vi "Labview_Database_write.vi"() -> ()   [LabVIEW 2012]
uses:
  <vilib>/addons/database/NI_Database_API.lvlib
  <vilib>/addons/database/Connection.llb/DB Tools Open Connec (Path).vi
  <vilib>/FieldPoint/Polymorphic Write.llb/FP Write (Float -IO).vi
  <vilib>/FieldPoint/Polymorphic Read.llb/FP Read (Float -IO).vi
  LabView ESIII/LabView ESIII/try.llb/Control 2.ctl
panel:
  out "current time":timestamp
  out "cFP-AI-112":dbl(graph)
  out "cFP-DO-401":dbl(graph)
  in  "Digital Output Switch":bool
  in  "sample data":T1={"String"="This is a test string", "Numeric"=101, "Numeric 2"=3.14} {"Numeric 2" format="%.2f"}
  out "tables":T2[](array[typedef])
  in  "stop":bool
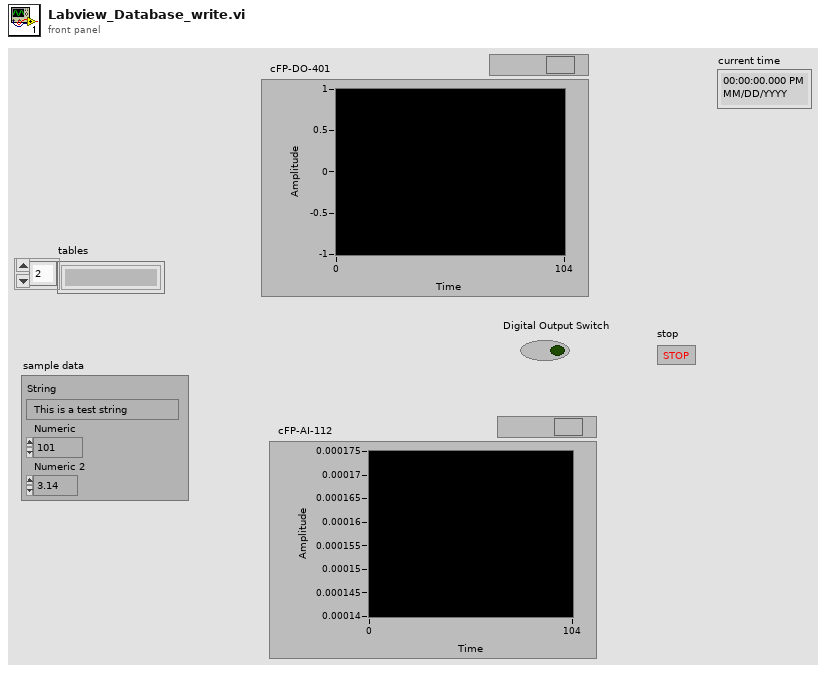
[diagram p1: front panel]
types:
  T1 = cluster{"String":string, "Numeric":i32, "Numeric 2":dbl}
  T2 = typedef "Control 2.ctl" = string
  T3 = typedef "NI_Database_API.lvlib/Conn ObjectReference.ctl" = refnum<k1>
  T4 = cluster{"date/time string":string, "value":dbl, "value":dbl}
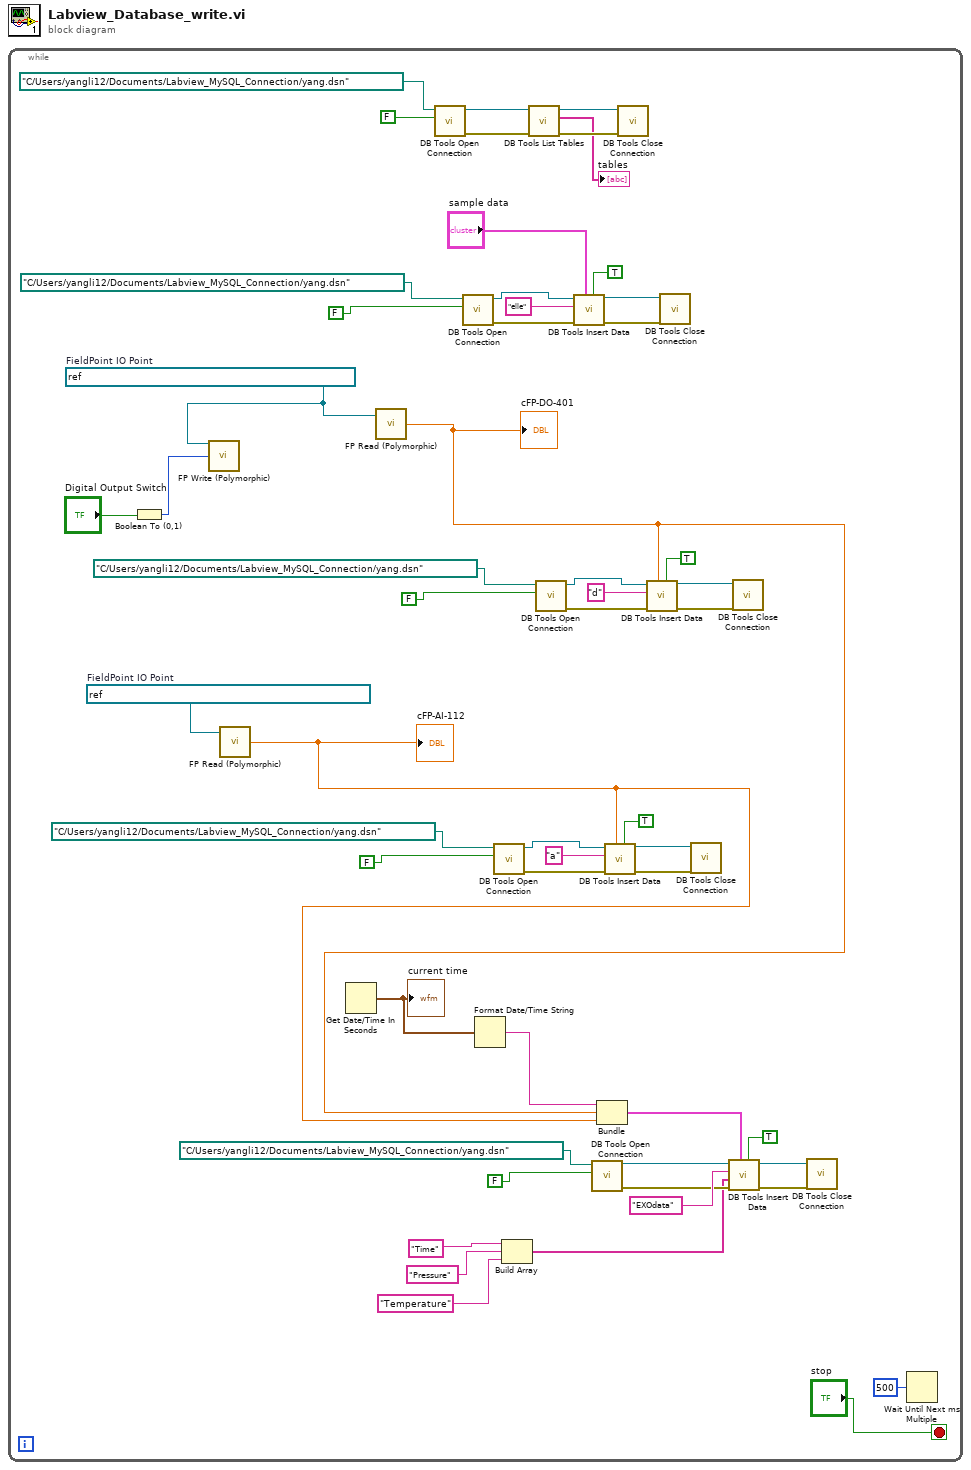
[diagram p0: block diagram]
diagram:
  n1 = while {
    stop <- "stop" stop-if-true
    w26 = refnum<k21> "FieldPoint\\Loomis434\\cFP-AI-112 @5\\Channel 0"  # FieldPoint IO Point
    w27 = refnum<k21> "FieldPoint\\Loomis434\\cFP-DO-401 @4\\Channel 0"  # FieldPoint IO Point
    n2 = Boolean To (0,1)(Boolean="Digital Output Switch") -> (0, 1=w28:i16)
    n3 = call-poly <vilib>:"FP Write (Polymorphic).vi"("FieldPoint IO Point In"=w27, "value"=w28) -> ()  [unwired: 11 in, 3 out]
    n4 = call-poly <vilib>:"FP Read (Polymorphic).vi"("FieldPoint IO Point In"=w26) -> ("value"=w10:dbl)  [unwired: 11 in, 3 out]
    "cFP-AI-112" <- w10
    n5 = Get Date/Time In Seconds() -> (seconds since 1Jan1904=w3:timestamp)
    "current time" <- w3
    n6 = call-poly <vilib>:"FP Read (Polymorphic).vi"("FieldPoint IO Point In"=w27) -> ("value"=w11:dbl)  [unwired: 11 in, 3 out]
    "cFP-DO-401" <- w11
    n7 = call-poly <vilib>:"DB Tools Open Connection.vi"("prompt? (F)"=FALSE, "connection information"=path "C:/Users/yangli12/Documents/Labview_MySQL_Connection/yang.dsn") -> ("error out"=w46:errorcluster, "connection reference"=w49:T3)  [unwired: 6 in]
    n8 = call-poly <vilib>:"DB Tools Open Connection.vi"("prompt? (F)"=FALSE, "connection information"=path "C:/Users/yangli12/Documents/Labview_MySQL_Connection/yang.dsn") -> ("error out"=w42:errorcluster, "connection reference"=w43:T3)  [unwired: 6 in]
    n9 = Format Date/Time String(seconds (now)=w3) -> (date/time string=w4:string)  [unwired: 2 in]
    n10 = call-poly <vilib>:"DB Tools Open Connection.vi"("prompt? (F)"=FALSE, "connection information"=path "C:/Users/yangli12/Documents/Labview_MySQL_Connection/yang.dsn") -> ("error out"=w20:errorcluster, "connection reference"=w21:T3)  [unwired: 6 in]
    n11 = Build Array("Time" ("table"), "Pressure" ("table"), "Temperature" ("table")) -> (w5:string[])
    n12 = call <vilib>:"DB Tools List Tables.vi"("error in (no error)"=w46, "connection reference"=w49) -> ("error out"=w53:errorcluster, "tables"=→"tables":string[], "connection reference out"=w54:T3)  [unwired: 3 in]
    n13 = call-poly <vilib>:"DB Tools Open Connection.vi"("prompt? (F)"=FALSE, "connection information"=path "C:/Users/yangli12/Documents/Labview_MySQL_Connection/yang.dsn") -> ("error out"=w32:errorcluster, "connection reference"=w33:T3)  [unwired: 6 in]
    n14 = call <vilib>:"DB Tools Insert Data.vi"("create table? (F)"=TRUE, "data"="sample data", "error in (no error)"=w42, "table"="elle", "connection reference"=w43) -> ("error out"=w47:errorcluster, "connection reference out"=w48:T3)  [unwired: 5 in]
    n15 = call-poly <vilib>:"DB Tools Open Connection.vi"("prompt? (F)"=FALSE, "connection information"=path "C:/Users/yangli12/Documents/Labview_MySQL_Connection/yang.dsn") -> ("error out"=w12:errorcluster, "connection reference"=w13:T3)  [unwired: 6 in]
    n16 = Bundle("date/time string"=w4, "value"=w11, "value"=w10) -> (w9:T4)  [unwired: 1 in]
    n17 = call <vilib>:"DB Tools Insert Data.vi"("create table? (F)"=TRUE, "data"=w10, "error in (no error)"=w20, "table"="a", "connection reference"=w21) -> ("error out"=w24:errorcluster, "connection reference out"=w25:T3)  [unwired: 5 in]
    n18 = call <vilib>:"DB Tools Close Connection.vi"("error in (no error)"=w53, "connection reference"=w54) -> ()  [unwired: 5 in, 1 out]
    n19 = call <vilib>:"DB Tools Insert Data.vi"("create table? (F)"=TRUE, "data"=w11, "error in (no error)"=w32, "table"="d", "connection reference"=w33) -> ("error out"=w36:errorcluster, "connection reference out"=w37:T3)  [unwired: 5 in]
    n20 = call <vilib>:"DB Tools Close Connection.vi"("error in (no error)"=w47, "connection reference"=w48) -> ()  [unwired: 5 in, 1 out]
    n21 = call <vilib>:"DB Tools Close Connection.vi"("error in (no error)"=w24, "connection reference"=w25) -> ()  [unwired: 5 in, 1 out]
    n22 = call <vilib>:"DB Tools Insert Data.vi"("create table? (F)"=TRUE, "data"=w9, "error in (no error)"=w12, "columns"=w5, "table"="EXOdata", "connection reference"=w13) -> ("error out"=w1:errorcluster, "connection reference out"=w2:T3)  [unwired: 4 in]
    n23 = call <vilib>:"DB Tools Close Connection.vi"("error in (no error)"=w36, "connection reference"=w37) -> ()  [unwired: 5 in, 1 out]
    n24 = call <vilib>:"DB Tools Close Connection.vi"("error in (no error)"=w1, "connection reference"=w2) -> ()  [unwired: 5 in, 1 out]
    n25 = Wait Until Next ms Multiple(millisecond multiple=u32 500) -> ()  [unwired: 1 out]
  }
